vi "Write ILC.vi"(10 "ILC":refnum<class "ILC.lvclass">, 11 "ILCDAC2 in":refnum<class "ILCDAC2.lvclass">) -> (3 "ILCDAC2 out":refnum<class "ILCDAC2.lvclass">)   [LabVIEW 2015]
uses:
  ILCDAC2.lvclass
  <userlib>/Common/ILC/ILC/ILC.lvclass
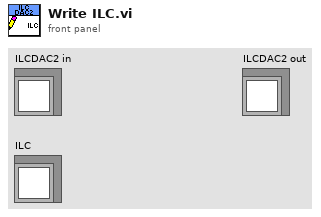
[diagram p1: front panel]
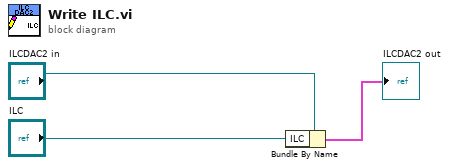
[diagram p0: block diagram]
diagram:
  n1 = Bundle By Name(cluster="ILCDAC2 in", "ILC"="ILC") -> (→"ILCDAC2 out":cluster{})
